vi "Remove Module from Project by Name.vi"(6 "TreeControl in":refnum<vi>, 8 "error in":errorcluster, 10 "Module Name":string, 11 "Data Cluster In":T1={"Project"=refnum, "Current Selection"={"Library"=refnum, "VI"=refnum}, "Module ID"=-1, "Tree Selection"=""}) -> (0 "error out":errorcluster, 3 "Data Cluster Out":T1={"Project"=refnum, "Current Selection"={"Library"=refnum, "VI"=refnum}, "Module ID"=-1, "Tree Selection"=""})   [LabVIEW 2020, in "Panther Dashboard.lvlib"]
doc: "Gets the Singleton and Cloneable references and creates a list of each type of DQMH Modules"
uses:
  Panther Dashboard.lvlib
  Module Data--cluster.ctl
  Class/Project/Project.lvclass
  C:/GitClones/PantherDashboard/src/LabVIEW/Panther Dashboard/Class/LabVIEWItem/LabVIEWItem.lvclass
  Class/Library/Library.lvclass
  Class/VI/VI.lvclass
  Class/Project/Project.lvclass/Project.ctl
  Class/LabVIEWItem/LabVIEWItem.lvclass/LabVIEWItem.ctl
  Class/Library/Library.lvclass/Library.ctl
  Class/LabVIEWItem/Read Item Name.vi
  Class/Library/Read Library Ref.vi
  Class/Project/Write Libraries.vi
  Class/LabVIEWItem/Read Item Tag.vi
  Class/Project/Read Libraries.vi
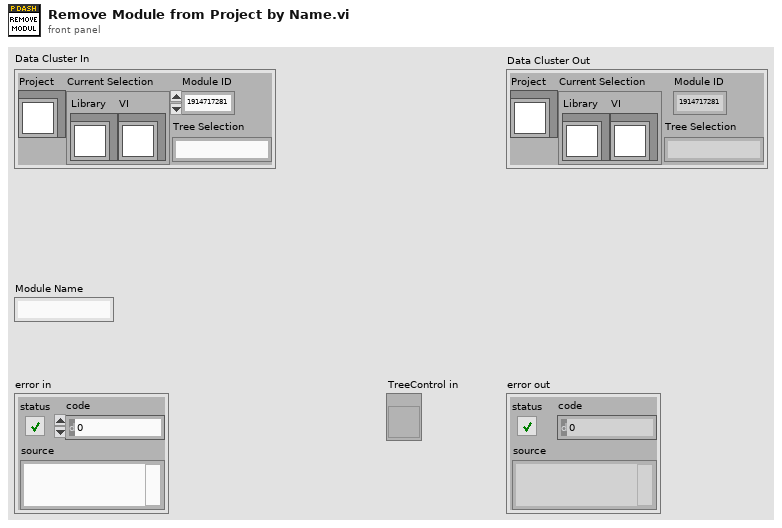
[diagram p1: front panel]
types:
  T1 = typedef "Panther Dashboard.lvlib/Module Data--cluster.ctl" = cluster{"Project":refnum<class "Project.lvclass">, "Current Selection":cluster{"Library":refnum<class "Library.lvclass">, "VI":refnum<class "VI.lvclass">}, "Module ID":i32, "Tree Selection":string}
  T2 = typedef "Tree Map.lvlib/Tree Map Data.ctl" = map{string, cluster{"Child Paths Set":set{string}, "Name":string, "Data":string, "Attributes":map{string, string}}}
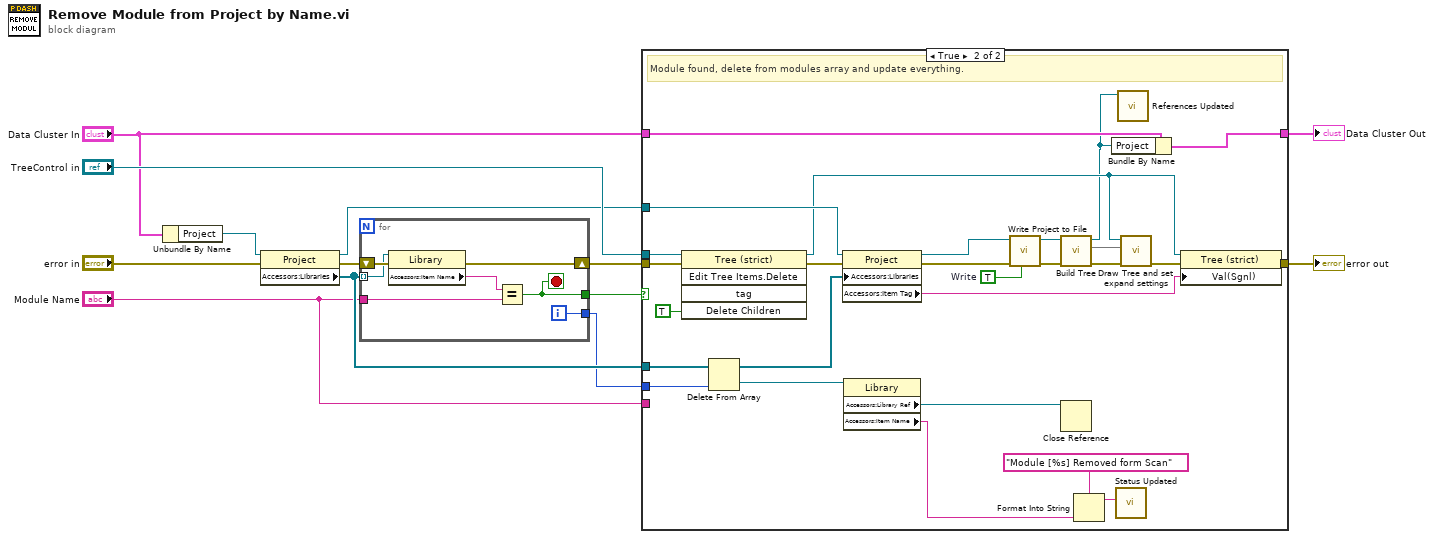
[diagram p0: block diagram]
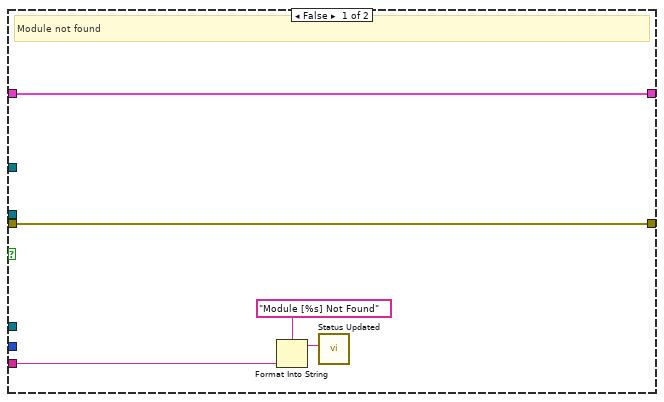
[diagram p2: hidden frame]
diagram:
  n1 = Unbundle By Name("Data Cluster In") -> ("Project"=w6:refnum<class "Project.lvclass">)
  n2 = property class="Project"(reference=w6, error in="error in") -> (reference out=w4:refnum<class "Project.lvclass">, error out=w13:errorcluster, "Accessors:Libraries"=w5:refnum<class "Library.lvclass">[])
  n3 = for {
    tunnel: w5 -> [w18] mode=indexing
    tunnel: [w17] -> w3
    shift-right: [w19] -> w11
    shift-left: w13 -> [w20]
    tunnel: "Module Name" -> [w15]
    tunnel: [w14] -> w2
    i -> [w17]
    stop <- w14 stop-if-true
    n4 = property class="Library"(reference=w18, error in=w20) -> (error out=w19:errorcluster, "Accessors:Item Name"=w16:string)  [unwired: 1 out]
    n5 = Equal?(x=w16, y=w15) -> (x = y?=w14:bool)
  }
  n6 = case shown="True" w2 {
    tunnel: w11 -> [w25 w52]
    tunnel: [w25 w49] -> w10
    tunnel: "TreeControl in" -> [_ w45]
    tunnel: "Data Cluster In" -> [w24 w40]
    tunnel: [w24 w39] -> w7
    tunnel: w5 -> [_ w38]
    tunnel: w4 -> [_ w35]
    tunnel: w3 -> [_ w28]
    tunnel: "Module Name" -> [w21 _]
    frame False {
      # "Module not found"
      n7 = Format Into String(format string="Module [%s] Not Found" ("Status"), w21) -> (resulting string=w22:string)  [unwired: 2 in, 1 out]
      n8 = call "Status Updated.vi"("Status"=w22) -> ()  [unwired: 10 in, 1 out]
    }
    frame True {
      w43 = TRUE  # Write
      # "Module found, delete from modules array and update everything."
      n9 = invoke class="Tree (strict)" method="Edit Tree Items.Delete"(reference=w45, error in=w52, "Delete Children"=TRUE ("Delete Children?")) -> (reference out=w33:refnum<vi>, error out=w51:errorcluster)  [unwired: 2 in, 3 out]
      n10 = Delete From Array "Delete From Array"(array=w38, index=w28) -> (deleted portion=w27:refnum<class "Library.lvclass">, array with subset deleted=w37:refnum<class "Library.lvclass">[])  [unwired: 1 in]
      n11 = property class="Project"(reference=w35, error in=w51, "Accessors:Libraries"=w37) -> (reference out=w31:refnum<class "Project.lvclass">, error out=w48:errorcluster, "Accessors:Item Tag"=w26:string)
      n12 = property class="Library"(reference=w27) -> ("Accessors:Library Ref"=w36:refnum<vi>, "Accessors:Item Name"=w29:string)  [unwired: 1 in, 2 out]
      n13 = call "Write Project to File.vi"("Write"=w43, "error in"=w48, "Project In"=w31) -> ("error out"=w47:errorcluster, "Project Out"=w30:refnum<class "Project.lvclass">)  [unwired: 6 in, 1 out]
      n14 = call "Build Tree.vi"("error in"=w47, "Project in"=w30) -> ("error out"=w50:errorcluster, "Tree Map Out"=w34:T2, "Project Out"=w32:refnum<class "Project.lvclass">)  [unwired: 7 in]
      n15 = Close Reference(reference=w36) -> ()  [unwired: 1 in, 1 out]
      n16 = Format Into String(format string="Module [%s] Removed form Scan" ("Status"), w29) -> (resulting string=w41:string)  [unwired: 2 in, 1 out]
      n17 = Bundle By Name(cluster=w40, "Project"=w32) -> (w39:T1)
      n18 = call "Status Updated.vi"("Status"=w41) -> ()  [unwired: 10 in, 1 out]
      n19 = call "References Updated.vi"("Project"=w32) -> ()  [unwired: 10 in, 1 out]
      n20 = call "Draw Tree and set expand settings.vi"("error in"=w50, "Tree Map In"=w34, "TreeControl in"=w33) -> ("error out"=w46:errorcluster)  [unwired: 8 in]
      n21 = property class="Tree (strict)"(reference=w33, error in=w46, "Val(Sgnl)"=w26) -> (error out=w49:errorcluster)  [unwired: 1 out]
    }
  }
  "error out" <- w10
  "Data Cluster Out" <- w7
